vi "Reset.vi"(8 "error in (no error)":errorcluster, 11 "Debug Log in":refnum<class "Debug Log.lvclass">) -> (0 "error out":errorcluster, 3 "Debug Log out":refnum<class "Debug Log.lvclass">)   [LabVIEW 2020, in "Debug Log.lvclass"]
uses:
  Debug Log.lvclass
  Debug Data/Debug Data.lvclass
  Debug Log.lvclass/Debug Log.ctl
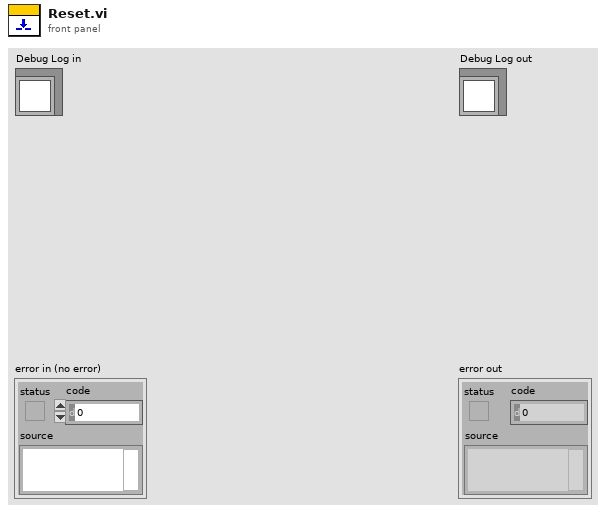
[diagram p1: front panel]
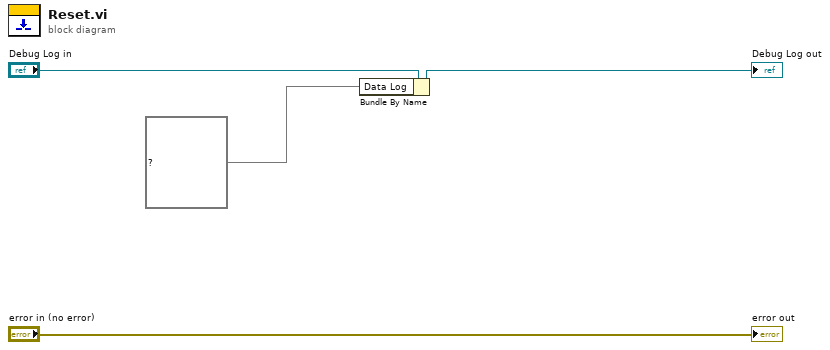
[diagram p0: block diagram]
diagram:
  n1 = Bundle By Name(cluster="Debug Log in", "Data Log"=map{u32, refnum<class "Debug Data.lvclass">} {}) -> (→"Debug Log out":refnum<class "Debug Log.lvclass">)
  "error out" <- "error in (no error)"
